vi "Init.vi"(8 "error in (no error)":errorcluster, 11 "Action Request":refnum<user-event>) -> (0 "error out":errorcluster, 3 "TimerActionController out":refnum<class "TimerActionController.lvclass">)   [LabVIEW 2020, in "Timer Demo.lvlib" / "TimerActionController.lvclass"]
uses:
  TimerActionController.lvclass
  Timer Action.ctl
  Timer Demo.lvlib
  Timer Action Response.ctl
  Timer Action Request.ctl
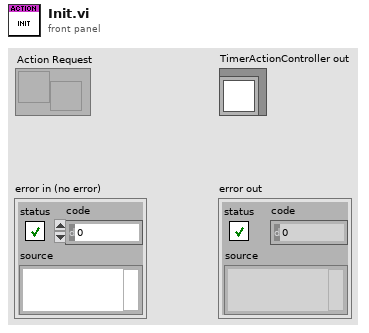
[diagram p1: front panel]
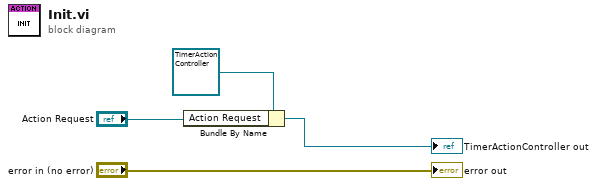
[diagram p0: block diagram]
diagram:
  n1 = Bundle By Name(cluster=refnum<class "TimerActionController.lvclass"> refnum ("TimerActionController in"), "Action Request"="Action Request") -> (→"TimerActionController out":refnum<class "TimerActionController.lvclass">)
  "error out" <- "error in (no error)"
